vi "[Map] Find Max Value.vi"(11 "Map":map{string, i32}(c390)) -> (2 "Max Value":i32, 3 "Key With Max Value":string)   [LabVIEW 2019]
doc: "This finds the maximum VALUE within a map and returns that value, along with the associated key."
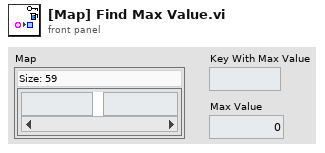
[diagram p1: front panel]
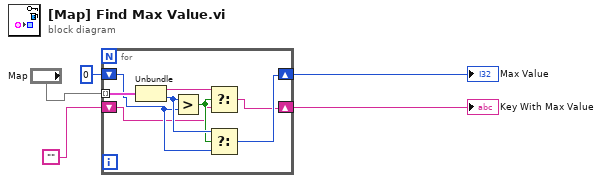
[diagram p0: block diagram]
diagram:
  n1 = for {
    tunnel: "Map" -> [w13] mode=indexing
    shift-right: [w10] -> w4
    shift-left: 0 -> [w11]
    shift-right: [w6] -> w5
    shift-left: "" -> [w7]
    n2 = Unbundle(w13) -> (w8:string, w12:i32)
    n3 = Greater?(x=w12, y=w11) -> (0:w9:bool)
    n4 = Select(t=w8, s=w9, f=w7) -> (s? t:f=w6:string)
    n5 = Select(t=w12, s=w9, f=w11) -> (s? t:f=w10:i32)
  }
  "Key With Max Value" <- w5
  "Max Value" <- w4
